vi "Peak Detect.vi"(7 "initialize":bool, 8 "Influence":dbl format="%#_13g", 9 "Diffs":dbl, 10 "Lag":i32=100, 11 "x":dbl) -> (3 "Peak?":bool)   [LabVIEW 2015]
uses:
  <vilib>/ptbypt/NI_PtbyPt.lvlib
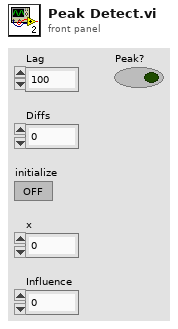
[diagram p1: front panel]
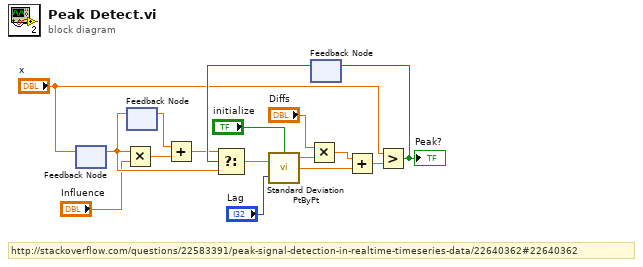
[diagram p0: block diagram]
diagram:
  # "http://stackoverflow.com/questions/22583391/peak-signal-detection-in-realtime-timeseries-data/22640362#22640362"
  n1 = feedback #1() -> (w12:dbl)  [unwired: 1 in]
  n2 = feedback-in #1("x") -> ()
  n3 = Multiply(x=w12, y="Influence") -> (x*y=w9:dbl)
  n4 = feedback #2() -> (w11:dbl)  [unwired: 1 in]
  n5 = feedback-in #2(w12) -> ()
  n6 = Add(x=w11, y=w9) -> (x+y=w10:dbl)
  n7 = feedback #3() -> (w15:bool)  [unwired: 1 in]
  n8 = Select(t=w10, s=w15, f=w12) -> (s? t:f=w8:dbl)
  n9 = call <vilib>:"Standard Deviation PtByPt.vi"("x"=w8, "sample length"="Lag", "initialize"="initialize") -> ("standard deviation"=w1:dbl, "mean"=w3:dbl)  [unwired: 1 out]
  n10 = Multiply(x="Diffs", y=w1) -> (x*y=w4:dbl)
  n11 = Add(x=w4, y=w3) -> (x+y=w5:dbl)
  n12 = Greater?(x="x", y=w5) -> (0:w14:bool)
  "Peak?" <- w14
  n13 = feedback-in #3(w14) -> ()
